vi "Load Ranges.vi"(8 "error in (no error)":errorcluster, 10 "Group":refnum<class "Group DBL.lvclass">, 11 "DiscreteRangeControl in":refnum<class "DiscreteRangeControl.lvclass">) -> (0 "error out":errorcluster, 3 "DiscreteRangeControl out":refnum<class "DiscreteRangeControl.lvclass">)   [LabVIEW 2020, in "VolatusControl.lvlib" / "DiscreteRangeControl.lvclass"]
uses:
  DiscreteRangeControl.lvclass
  lv-vecto/Vecto/Group DBL/Group DBL.lvclass
  C:/dev/lv20CE/relink/lv-vecto/Vecto/Group/Group.lvclass
  DiscreteRangeControl.lvclass/DiscreteRangeControl.ctl
  lv-cdm/CDM-Config/Config Element/Owner.vi
  lv-cdm/CDM-Config/Config Manager/Lookup Descendant.vi
  lv-cdm/CDM-Config/Config Element/Config Element.lvclass
  lv-cdm/CDM-Config/Config Filter/Config Lookup.lvclass
  lv-vecto/Vecto/Group/Group.lvclass
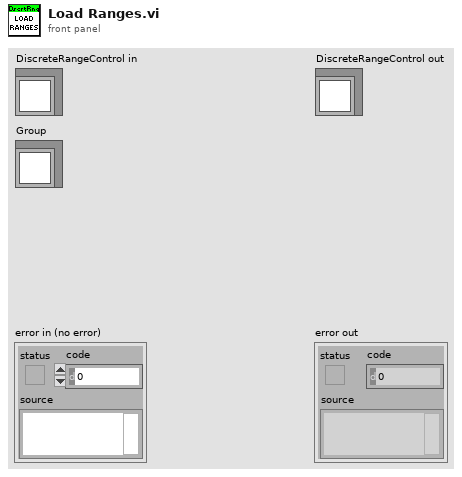
[diagram p1: front panel]
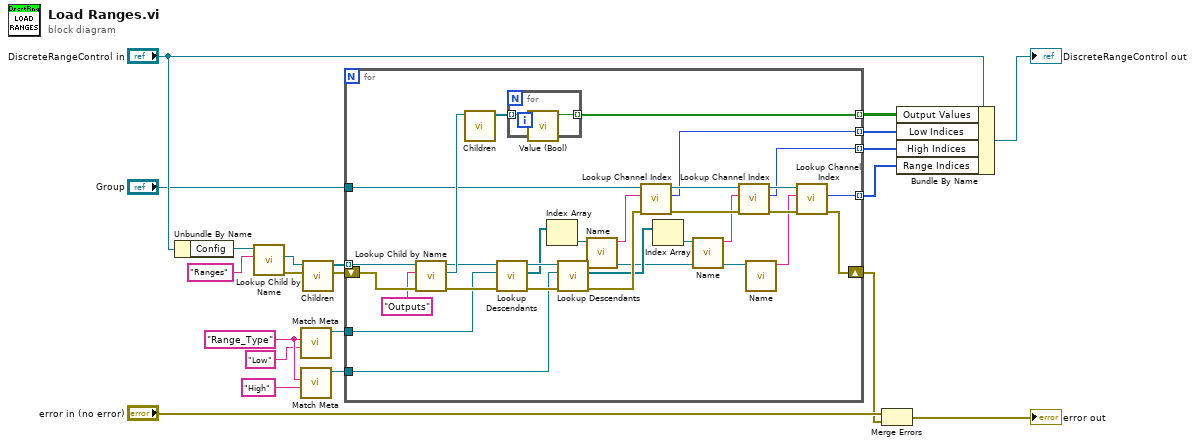
[diagram p0: block diagram]
diagram:
  w12 = "Range_Type" ("Name")
  n1 = Unbundle By Name("DiscreteRangeControl in") -> ("Config"=w19:refnum<class "Config Element.lvclass">)
  n2 = call "Lookup Child by Name.vi"("Name"="Ranges", "Config Element in"=w19) -> ("error out"=w17:errorcluster, "Child"=w16:refnum<class "Config Element.lvclass">)  [unwired: 6 in, 2 out]
  n3 = call "Match Meta.vi"("Value (Any)"="Low" ("Name"), "Name"=w12) -> ("Config Lookup out"=w10:refnum<class "Config Lookup.lvclass">)  [unwired: 8 in, 1 out]
  n4 = call "Match Meta.vi"("Value (Any)"="High" ("Name"), "Name"=w12) -> ("Config Lookup out"=w9:refnum<class "Config Lookup.lvclass">)  [unwired: 8 in, 1 out]
  n5 = call "Children.vi"("error in (no error)"=w17, "Config Element in"=w16) -> ("error out"=w14:errorcluster, "Elements"=w15:refnum<class "Config Element.lvclass">[])  [unwired: 8 in]
  n6 = for {
    tunnel: w15 -> [w49] mode=indexing
    shift-right: [w25] -> w6
    shift-left: w14 -> [w48]
    tunnel: w10 -> [w39]
    tunnel: w9 -> [w38]
    tunnel: "Group" -> [w36]
    tunnel: [w26] -> w4 mode=indexing
    tunnel: [w24] -> w3 mode=indexing
    tunnel: [w23] -> w2 mode=indexing
    tunnel: [w22] -> w1 mode=indexing
    n7 = call "Lookup Child by Name.vi"("error in (no error)"=w48, "Name"="Outputs", "Config Element in"=w49) -> ("error out"=w43:errorcluster, "Child"=w46:refnum<class "Config Element.lvclass">, "Config Element out"=w44:refnum<class "Config Element.lvclass">)  [unwired: 5 in, 1 out]
    n8 = call "Children.vi"("Config Element in"=w46) -> ("Elements"=w45:refnum<class "Config Element.lvclass">[])  [unwired: 9 in, 1 out]
    n9 = call "Lookup Descendants.vi"("error in (no error)"=w43, "Lookup"=w39, "Config Element in"=w44) -> ("error out"=w41:errorcluster, "Descendants"=w40:refnum<class "Config Element.lvclass">[], "Config Element out"=w42:refnum<class "Config Element.lvclass">)  [unwired: 6 in]
    n10 = for {
      tunnel: w45 -> [w53] mode=indexing
      tunnel: [w52] -> w24 mode=indexing
      n11 = call "Value (Bool).vi"("Config Element in"=w53) -> ("Bool Value"=w52:bool)  [unwired: 9 in, 1 out]
    }
    n12 = Index Array(array=w40) -> (element=w37:refnum<class "Config Element.lvclass">)  [unwired: 1 in]
    n13 = call "Lookup Descendants.vi"("error in (no error)"=w41, "Lookup"=w38, "Config Element in"=w42) -> ("error out"=w34:errorcluster, "Descendants"=w31:refnum<class "Config Element.lvclass">[], "Config Element out"=w29:refnum<class "Config Element.lvclass">)  [unwired: 6 in]
    n14 = call "Name.vi"("Config Element in"=w37) -> ("Name"=w35:string)  [unwired: 9 in, 1 out]
    n15 = call "Lookup Channel Index.vi"("error in (no error)"=w34, "Channel Name"=w35, "Group in"=w36) -> ("error out"=w50:errorcluster, "Index"=w23:i32, "Group out"=w30:refnum<class "Group DBL.lvclass">)  [unwired: 6 in]
    n16 = Index Array(array=w31) -> (element=w32:refnum<class "Config Element.lvclass">)  [unwired: 1 in]
    n17 = call "Name.vi"("Config Element in"=w32) -> ("Name"=w33:string)  [unwired: 9 in, 1 out]
    n18 = call "Lookup Channel Index.vi"("error in (no error)"=w50, "Channel Name"=w33, "Group in"=w30) -> ("error out"=w51:errorcluster, "Index"=w22:i32, "Group out"=w27:refnum<class "Group DBL.lvclass">)  [unwired: 6 in]
    n19 = call "Name.vi"("Config Element in"=w29) -> ("Name"=w28:string)  [unwired: 9 in, 1 out]
    n20 = call "Lookup Channel Index.vi"("error in (no error)"=w51, "Channel Name"=w28, "Group in"=w27) -> ("error out"=w25:errorcluster, "Index"=w26:i32)  [unwired: 6 in, 1 out]
  }
  n21 = Merge Errors("error in (no error)", w6) -> (→"error out":errorcluster)
  n22 = Bundle By Name(cluster="DiscreteRangeControl in", "Output Values"=w3, "Low Indices"=w2, "High Indices"=w1, "Range Indices"=w4) -> (→"DiscreteRangeControl out":refnum<class "DiscreteRangeControl.lvclass">)
